vi "Sum Positive Array Elements.vi"(4 "Array":dbl[](array[numeric])) -> (1 "Positive Element Sum":dbl)   [LabVIEW 2013]
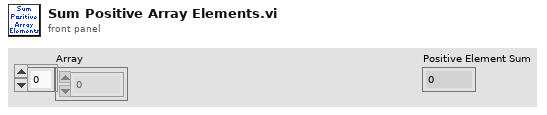
[diagram p1: front panel]
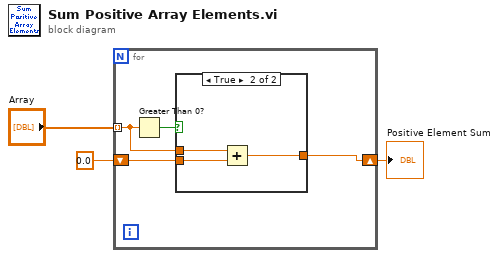
[diagram p0: block diagram]
diagram:
  n1 = for {
    shift-right: [w4] -> w1
    shift-left: 0.0 -> [w6]
    tunnel: "Array" -> [w5] mode=indexing
    n2 = Greater Than 0?(x=w5) -> (x > 0?=w7:bool)
    n3 = case shown="True" w7 {
      tunnel: w6 -> [w8 w11]
      tunnel: w5 -> [_ w10]
      tunnel: [w8 w9] -> w4
      frame False {
      }
      frame True {
        n4 = Add(x=w10, y=w11) -> (x+y=w9:dbl)
      }
    }
  }
  "Positive Element Sum" <- w1
